vi "test Triggered Acyclic Frame.vi"(8 "error in":errorcluster, 11 "Loopback in":refnum<class "Loopback.lvclass">) -> (0 "error out":errorcluster, 3 "Loopback out":refnum<class "Loopback.lvclass">)   [LabVIEW 2020, in "Loopback.lvclass"]
uses:
  Loopback.lvclass
  C:/Program Files (x86)/National Instruments/LabVIEW 2020/vi.lib/addons/_JKI Toolkits/VI Tester/TestCase.llb/TestCase.lvclass
  niveristand-custom-device-testing-tools/VeriStandTestUtilities/VeriStandTestUtilities.lvlib
  <vilib>/NI VeriStand/Execution/Workspace/NI_VS Workspace ExecutionAPI.lvlib
  <vilib>/NI VeriStand/Execution/Workspace/NI VeriStand - Set Single Channel Value.vi
  <vilib>/addons/_JKI Toolkits/VI Tester/TestCase.llb/TestCase.lvclass
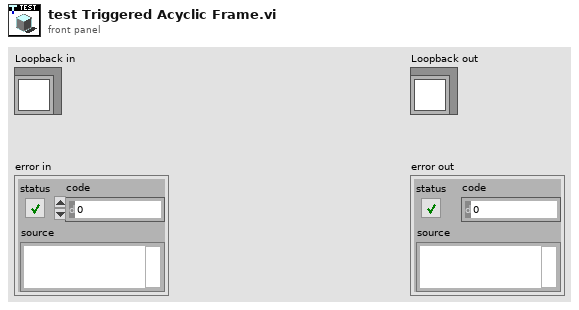
[diagram p1: front panel]
types:
  T1 = typedef "NI_VS Workspace ExecutionAPI.lvlib/WorkspaceAPI.ctl" = refnum<k24>
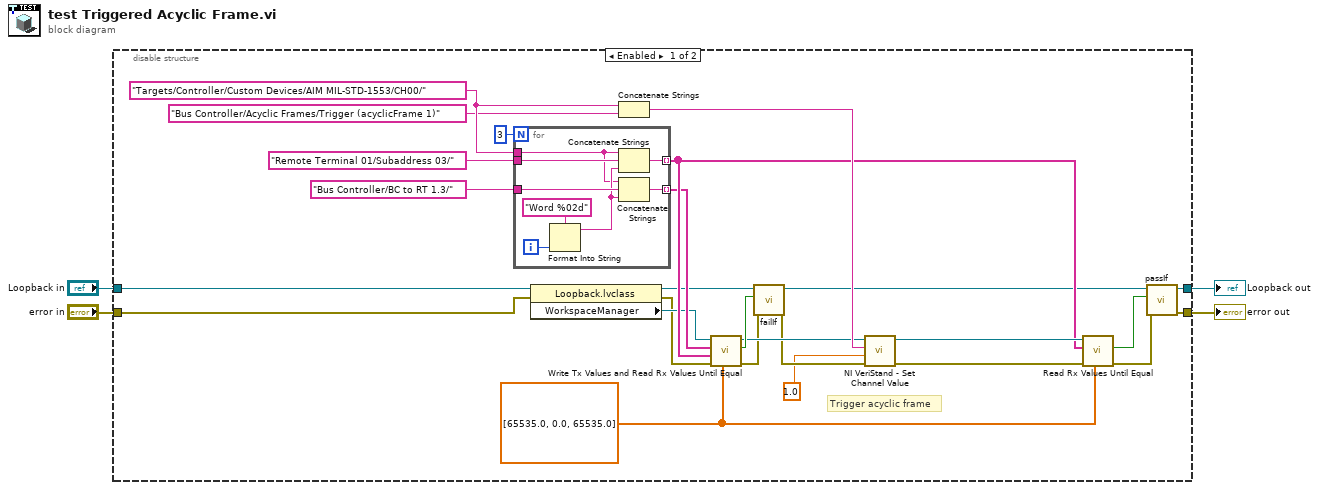
[diagram p0: block diagram]
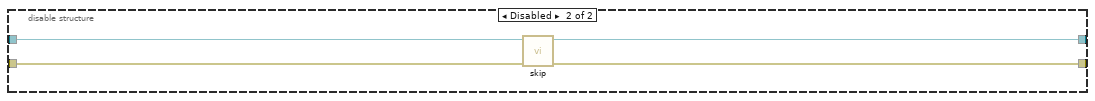
[diagram p2: hidden frame]
diagram:
  n1 = disable-structure shown="Enabled" {
    disable-tunnel: [w29 w40] -> w4
    disable-tunnel: [w28 w39] -> w3
    disable-tunnel: "Loopback in" -> [w8 w41]
    disable-tunnel: "error in" -> [w7 w42]
    frame Enabled {
      w30 = "Targets/Controller/Custom Devices/AIM MIL-STD-1553/CH00/" ("base name for channel aliases")
      w25 = dbl[] [65535.0, 0.0, 65535.0]
      # "Trigger acyclic frame"
      n2 = for {
        N: 3 -> [_]
        tunnel: "Bus Controller/BC to RT 1.3/" ("Channel") -> [w37]
        tunnel: [w38] -> w16 mode=indexing
        tunnel: "Remote Terminal 01/Subaddress 03/" ("Channel") -> [w36]
        tunnel: [w35] -> w18 mode=indexing
        tunnel: w30 -> [w31]
        i -> [w34]
        n3 = Format Into String(format string="Word %02d", w34) -> (resulting string=w33:string)  [unwired: 2 in, 1 out]
        n4 = Concatenate Strings(w31, w36, w33) -> (w35:string)
        n5 = Concatenate Strings(w31, w37, w33) -> (w38:string)
      }
      n6 = property class="Loopback.lvclass"(reference=w8, error in=w7) -> (reference out=w5:refnum<class "Loopback.lvclass">, error out=w6:errorcluster, "WorkspaceManager"=w9:T1)
      n7 = Concatenate Strings(w30, "Bus Controller/Acyclic Frames/Trigger (acyclicFrame 1)") -> (w27:string)
      n8 = call "Write Tx Values and Read Rx Values Until Equal.vi"("Tx values"=w25, "error in"=w6, "Rx aliases"=w18, "Tx aliases"=w16, "workspace manager in"=w9) -> ("error out"=w17:errorcluster, "values equal"=w24:bool, "workspace manager out"=w20:T1)  [unwired: 4 in]
      n9 = call-dynamic "failIf.vi"("error in (no error)"=w17, "fail"=w24, "TestCase in"=w5) -> ("error out"=w14:errorcluster, "TestCase out"=w15:refnum<class "Loopback.lvclass">)  [unwired: 7 in]
      n10 = call-poly <vilib>:"NI VeriStand - Set Channel Value.vi"("error in (no error)"=w14, "Value"=1.0, "Channel"=w27, "WorkspaceManager in"=w20) -> ("error out"=w23:errorcluster, "WorkspaceManager out"=w22:T1)  [unwired: 6 in]
      n11 = call "Read Rx Values Until Equal.vi"("expected values"=w25, "error in"=w23, "Rx aliases"=w18, "workspace manager in"=w22) -> ("error out"=w21:errorcluster, "values equal expected"=w19:bool)  [unwired: 5 in, 1 out]
      n12 = call-dynamic "passIf.vi"("error in (no error)"=w21, "pass"=w19, "TestCase in"=w15) -> ("error out"=w29:errorcluster, "TestCase out"=w28:refnum<class "Loopback.lvclass">)  [unwired: 7 in]
    }
    frame Disabled {
      n13 = call <vilib>:"skip.vi"("error in (no error)"=w42, "TestCase in"=w41) -> ("error out"=w40:errorcluster, "TestCase out"=w39:refnum<class "Loopback.lvclass">)  [unwired: 8 in]
    }
  }
  "error out" <- w4
  "Loopback out" <- w3
